vi "Set Subroutine Info.vi"(0 "subroutine in":string, 11 "error in":errorcluster) -> (15 "error out":errorcluster)   [LabVIEW 2021, in "Converter Reusables.lvlib"]
uses:
  Converter Reusables.lvlib
  TypeDefs/Dictionary States.ctl
  TypeDefs/Error Information.ctl
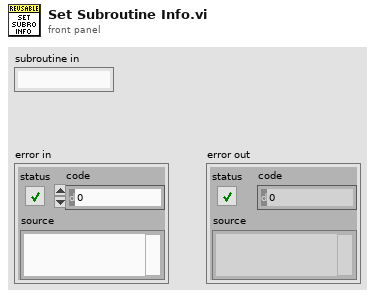
[diagram p1: front panel]
types:
  T1 = typedef "Converter Reusables.lvlib/Error Information.ctl" = cluster{"subroutine":string, "error data":errorcluster}
  T2 = typedef "Converter Reusables.lvlib/Dictionary States.ctl" = enum16{"Set", "Get", "Delete", "Delete All"}
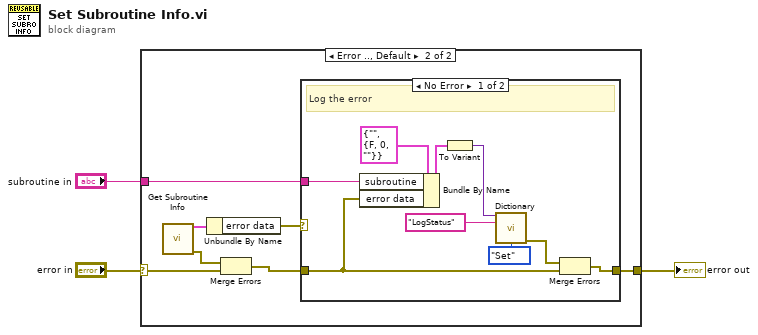
[diagram p0: block diagram]
diagram:
  n1 = case shown="Error .., Default" "error in" {
    selector: "error in" -> [w4 w10]
    tunnel: "subroutine in" -> [_ w11]
    tunnel: [w4 w7] -> w1
    frame No Error {
    }
    frame Error, Default {
      n2 = call "Get Subroutine Info.vi"() -> ("data"=w9:T1, "error out"=w5:errorcluster)  [unwired: 14 in]
      n3 = Unbundle By Name(w9) -> ("error data"=w8:errorcluster)
      n4 = Merge Errors(w5, w10) -> (w6:errorcluster)
      n5 = case shown="No Error" w8 {
        tunnel: w11 -> [w15 _]
        tunnel: w6 -> [w14 w21]
        tunnel: [w13 w21] -> w7
        frame No Error {
          # "Log the error"
          n6 = Bundle By Name(cluster=T1 {"subroutine"="", "error data"={"status"=FALSE, "code"=0, "source"=""}} ("ErrorInformation"), "subroutine"=w15, "error data"=w14) -> (w16:T1)
          n7 = To Variant(anything=w16) -> (Variant=w18:variant)
          n8 = call "Dictionary.vi"("variant in"=w18, "key"="LogStatus" ("Key"), "dict states"=Dictionary_States."Set" ("Dict States")) -> ("error out"=w12:errorcluster)  [unwired: 11 in, 1 out]
          n9 = Merge Errors(w12, w14) -> (w13:errorcluster)
        }
        frame Error {
          # "Pass the existing error information"
        }
      }
    }
  }
  "error out" <- w1
